vi "endOfBuffer.vi"(8 "error in (no error)":errorcluster, 11 "ModbusBuffer in":refnum<class "ModbusBufferBuilder.lvclass">) -> (0 "error out":errorcluster, 2 "EndOfBuffer":bool, 3 "ModbusBuffer out":refnum<class "ModbusBufferBuilder.lvclass">)   [LabVIEW 2016, in "ModbusBufferBuilder.lvclass"]
uses:
  ModbusBufferBuilder.lvclass
  ModbusBufferBuilder.lvclass/ModbusBufferBuilder.ctl
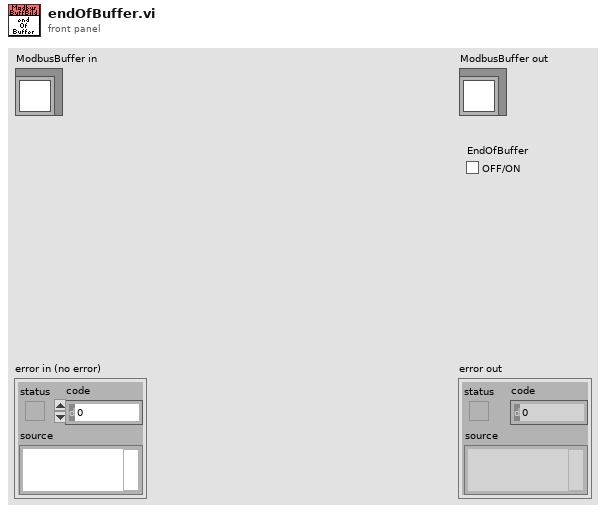
[diagram p1: front panel]
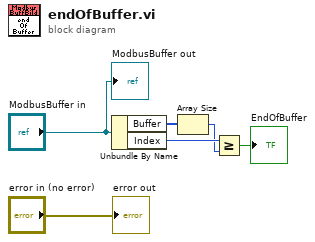
[diagram p0: block diagram]
diagram:
  n1 = Unbundle By Name("ModbusBuffer in") -> ("Buffer"=w4:u16[], "Index"=w6:i32)
  n2 = Array Size(array=w4) -> (size(s)=w5:i32)
  n3 = Greater Or Equal?(x=w6, y=w5) -> (x >= y?=→"EndOfBuffer":bool)
  "error out" <- "error in (no error)"
  "ModbusBuffer out" <- "ModbusBuffer in"
